vi "IRISS_FPGA_IO_v2.vi"() -> ()   [LabVIEW 2010]
doc: "This VI contains a basic quadrature decoder which is reset asynchronously upon clicking the reset button."
uses:
  <vilib>/platform/TimedLoop/XDataNode/XDataNode.xnode
  <vilib>/Platform/TimedLoop/XDataNode/nitl_modes.ctl
  <vilib>/Platform/TimedLoop/XDataNode/XDNodeRunTimeDep.lvlib
  <vilib>/Platform/TimedLoop/XDataNode/wakeup.ctl
  <vilib>/Platform/TimedLoop/XDataNode/timing_clust.ctl
  <vilib>/eio/EIONode/EIONode.xnode
  Library/KevinLibraryAll/labview/KevLib01.lvlib
panel:
  out "Home L4":bool
  out "Home L1":bool
  out "Home L2":bool
  out "Home L3":bool
  in  "Positive Direction C1-4":bool
  out "JumpBy2Error C1-4":i16
  out "32 bit Position C1-4":i32
  in  "Reset C1-4":bool
  in  "Positive Direction C1-1":bool
  out "JumpBy2Error C1-1":i16
  out "32 bit Position C1-1":i32
  in  "Reset C1-1":bool
  out "32 bit Position 17":i32
  in  "Reset 17":bool
  in  "Positive Direction 17":bool
  out "JumpBy2Error 17":i16
  out "32 bit Position 16":i32
  in  "Reset 16":bool
  in  "Positive Direction 16":bool
  out "JumpBy2Error 16":i16
  out "32 bit Position 15":i32
  in  "Reset 15":bool
  in  "Positive Direction 15":bool
  out "JumpBy2Error 15":i16
  out "32 bit Position 14":i32
  in  "Reset 14":bool
  in  "Positive Direction 14":bool
  out "JumpBy2Error 14":i16
  out "32 bit Position 13":i32
  in  "Reset 13":bool
  in  "Positive Direction 13":bool
  out "JumpBy2Error 13":i16
  out "32 bit Position 12":i32
  in  "Reset 12":bool
  in  "Positive Direction 12":bool
  out "JumpBy2Error 12":i16
  out "32 bit Position 11":i32
  in  "Reset 11":bool
  in  "Positive Direction 11":bool
  out "JumpBy2Error 11":i16
  out "32 bit Position 10":i32
  in  "Reset 10":bool
  in  "Positive Direction 10":bool
  out "JumpBy2Error 10":i16
  out "32 bit Position 9":i32
  in  "Reset 9":bool
  in  "Positive Direction 9":bool
  out "JumpBy2Error 9":i16
  out "JumpBy2Error 3":i16
  in  "Positive Direction 3":bool
  out "JumpBy2Error 1":i16
  in  "Positive Direction 1":bool
  out "AI":i16[](array[numeric])
  out "32 bit Position 3":i32
  in  "Reset 3":bool
  in  "AO":i16[](array[numeric])=[0, 0, 0, 0, 0, 0, 0, 0]
  out "32 bit Position 1":i32
  in  "Reset 1":bool
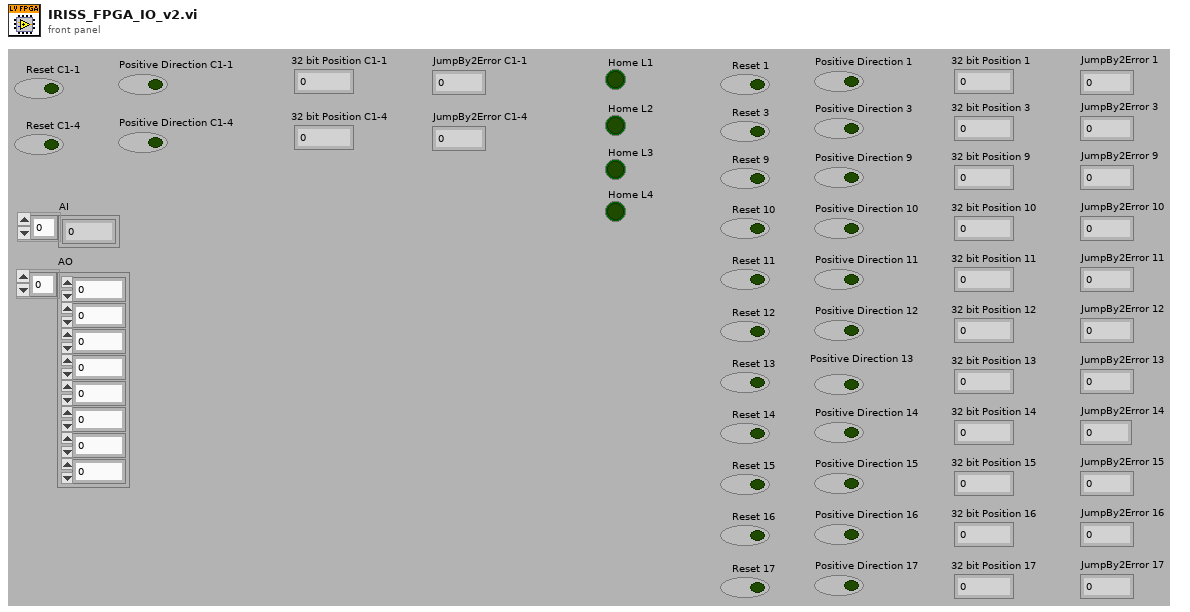
[diagram p1: front panel]
types:
  T1 = typedef "XDNodeRunTimeDep.lvlib/timing_clust.ctl" = cluster{"Expected End [f-1]":u64, "Actual End [f-1]":u64, "Finished Late? [f-1]":bool, "Expected End [i-1]":u64, "Actual End [i-1]":u64, "Finished Late? [i-1]":bool, "Expected Start [i]":u64, "Actual Start [i]":u64, "Expected Start [f]":u64, "Actual Start [f]":u64, "Source Name":string, "Structure Name":string, "Period":i64, "Deadline":i64, "Offset":i64, "Start":i64, "Priority":i32, "Timeout":i32, "Mode":T2, "Wakeup Reason":T3, "Error":errorcluster, "Source Type":string, "Secondary Source Type":string, "Global End Time":u64, "Global Start Time":u64, "Frame Duration":u64, "Iteration Duration":u64, "Assigned CPU":i32, "I/O Scan Engine Mode":u32}
  T2 = typedef "XDNodeRunTimeDep.lvlib/nitl_modes.ctl" = enum32{"No Change", "Process missed periods, maintain original phase", "Discard missed periods, maintain original phase", "Process missed periods, ignore original phase", "Discard missed periods, ignore original phase"}
  T3 = typedef "XDNodeRunTimeDep.lvlib/wakeup.ctl" = enum32{"Normal", "Aborted", "Asynchronous wakeup", "Timing source error", "Timed loop error", "Timeout"}
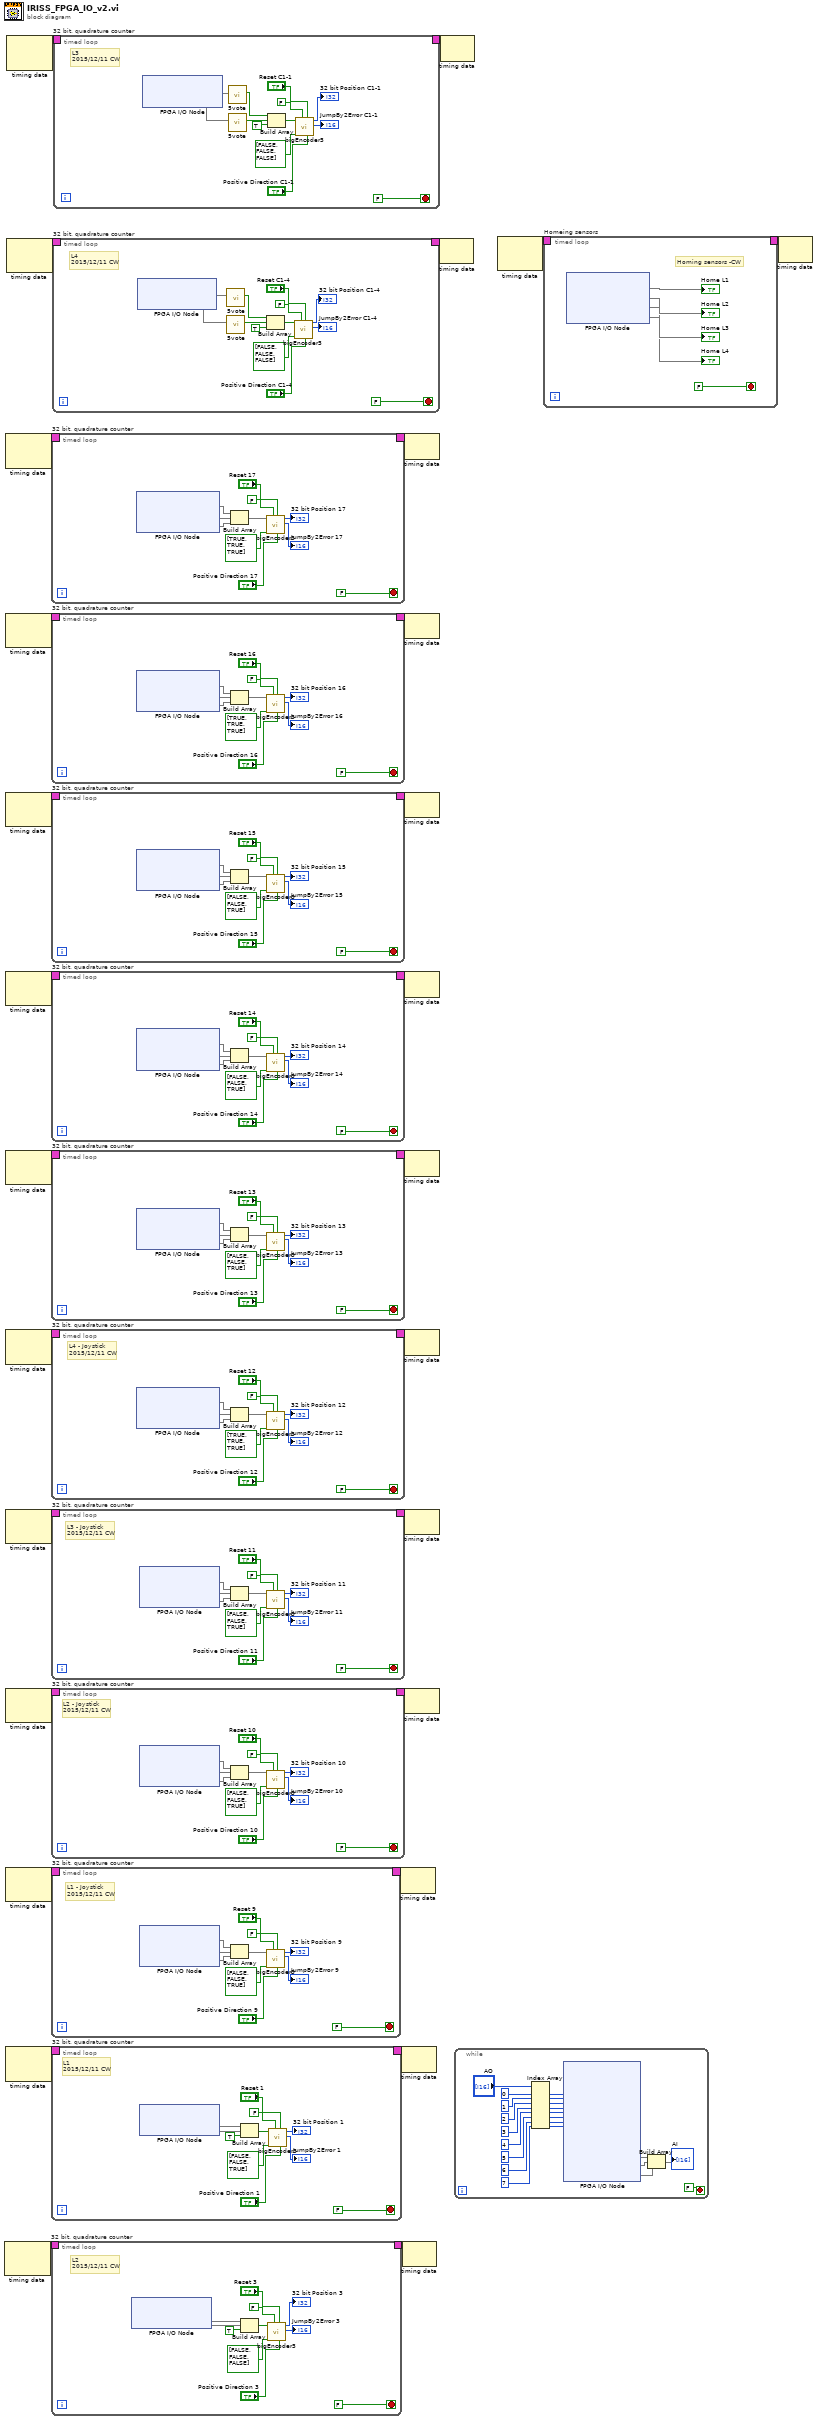
[diagram p0: block diagram]
diagram:
  n1 = node-c288() -> (w26:T1)  [unwired: 2 out]
  n2 = node-c288() -> (w8:T1)  [unwired: 2 out]
  n3 = node-c288() -> (w10:T1)  [unwired: 2 out]
  n4 = node-c288() -> (w12:T1)  [unwired: 2 out]
  n5 = node-c288() -> (w14:T1)  [unwired: 2 out]
  n6 = node-c288() -> (w16:T1)  [unwired: 2 out]
  n7 = node-c288() -> (w18:T1)  [unwired: 2 out]
  n8 = node-c288() -> (w20:T1)  [unwired: 2 out]
  n9 = node-c288() -> (w22:T1)  [unwired: 2 out]
  n10 = node-c288() -> (w24:T1)  [unwired: 2 out]
  n11 = node-c288() -> (w27:T1)  [unwired: 2 out]
  n12 = node-c288() -> (w4:T1)  [unwired: 2 out]
  n13 = node-c288() -> (w6:T1)  [unwired: 2 out]
  n14 = timed-loop "32 bit, quadrature counter" {
    timing-out: [_] -> w25
    timing: w26 -> [_]
    stop <- FALSE stop-if-true
    # "L2\n2015/12/11 CW"
    n15 = xnode "FPGA I/O Node"() -> ("Connector0/DIO2"=w32, "Connector0/DIO3"=w31)  [unwired: 2 in, 2 out]
    n16 = Build Array(w32, w31, TRUE ("element")) -> (w38:bool[])
    n17 = call "bigEncoder3.vi"("Positive Direction"="Positive Direction 3", "ForceReset"="Reset 3", "Allow C Reset?"=FALSE, "Reset Array"=bool[] [FALSE, FALSE, FALSE], "Encoder Array"=w38) -> ("JumpBy2Error"=→"JumpBy2Error 3":i16, "Position"=→"32 bit Position 3":i32)  [unwired: 5 out]
  }
  n18 = timed-loop "32 bit, quadrature counter" {
    timing-out: [_] -> w7
    timing: w8 -> [_]
    stop <- FALSE stop-if-true
    n19 = xnode "FPGA I/O Node"() -> ("Connector2/DIO24"=w51, "Connector2/DIO25"=w50, "Connector2/DIO26"=w42)  [unwired: 3 in, 3 out]
    n20 = Build Array(w51, w50, w42) -> (w49:void[])
    n21 = call "bigEncoder3.vi"("Positive Direction"="Positive Direction 17", "ForceReset"="Reset 17", "Allow C Reset?"=FALSE, "Reset Array"=bool[] [TRUE, TRUE, TRUE], "Encoder Array"=w49) -> ("JumpBy2Error"=→"JumpBy2Error 17":i16, "Position"=→"32 bit Position 17":i32)  [unwired: 5 out]
  }
  n22 = timed-loop "32 bit, quadrature counter" {
    timing-out: [_] -> w9
    timing: w10 -> [_]
    stop <- FALSE stop-if-true
    n23 = xnode "FPGA I/O Node"() -> ("Connector2/DIO21"=w64, "Connector2/DIO22"=w63, "Connector2/DIO23"=w55)  [unwired: 3 in, 3 out]
    n24 = Build Array(w64, w63, w55) -> (w62:void[])
    n25 = call "bigEncoder3.vi"("Positive Direction"="Positive Direction 16", "ForceReset"="Reset 16", "Allow C Reset?"=FALSE, "Reset Array"=bool[] [TRUE, TRUE, TRUE], "Encoder Array"=w62) -> ("JumpBy2Error"=→"JumpBy2Error 16":i16, "Position"=→"32 bit Position 16":i32)  [unwired: 5 out]
  }
  n26 = timed-loop "32 bit, quadrature counter" {
    timing-out: [_] -> w11
    timing: w12 -> [_]
    stop <- FALSE stop-if-true
    n27 = xnode "FPGA I/O Node"() -> ("Connector2/DIO18"=w77, "Connector2/DIO19"=w76, "Connector2/DIO20"=w68)  [unwired: 3 in, 3 out]
    n28 = Build Array(w77, w76, w68) -> (w75:void[])
    n29 = call "bigEncoder3.vi"("Positive Direction"="Positive Direction 15", "ForceReset"="Reset 15", "Allow C Reset?"=FALSE, "Reset Array"=bool[] [FALSE, FALSE, TRUE], "Encoder Array"=w75) -> ("JumpBy2Error"=→"JumpBy2Error 15":i16, "Position"=→"32 bit Position 15":i32)  [unwired: 5 out]
  }
  n30 = timed-loop "32 bit, quadrature counter" {
    timing-out: [_] -> w13
    timing: w14 -> [_]
    stop <- FALSE stop-if-true
    n31 = xnode "FPGA I/O Node"() -> ("Connector2/DIO15"=w90, "Connector2/DIO16"=w89, "Connector2/DIO17"=w81)  [unwired: 3 in, 3 out]
    n32 = Build Array(w90, w89, w81) -> (w88:void[])
    n33 = call "bigEncoder3.vi"("Positive Direction"="Positive Direction 14", "ForceReset"="Reset 14", "Allow C Reset?"=FALSE, "Reset Array"=bool[] [FALSE, FALSE, TRUE], "Encoder Array"=w88) -> ("JumpBy2Error"=→"JumpBy2Error 14":i16, "Position"=→"32 bit Position 14":i32)  [unwired: 5 out]
  }
  n34 = timed-loop "32 bit, quadrature counter" {
    timing-out: [_] -> w15
    timing: w16 -> [_]
    stop <- FALSE stop-if-true
    n35 = xnode "FPGA I/O Node"() -> ("Connector2/DIO12"=w103, "Connector2/DIO13"=w102, "Connector2/DIO14"=w94)  [unwired: 3 in, 3 out]
    n36 = Build Array(w103, w102, w94) -> (w101:void[])
    n37 = call "bigEncoder3.vi"("Positive Direction"="Positive Direction 13", "ForceReset"="Reset 13", "Allow C Reset?"=FALSE, "Reset Array"=bool[] [FALSE, FALSE, TRUE], "Encoder Array"=w101) -> ("JumpBy2Error"=→"JumpBy2Error 13":i16, "Position"=→"32 bit Position 13":i32)  [unwired: 5 out]
  }
  n38 = timed-loop "32 bit, quadrature counter" {
    timing-out: [_] -> w17
    timing: w18 -> [_]
    stop <- FALSE stop-if-true
    # "L4 - Joystick\n2015/12/11 CW"
    n39 = xnode "FPGA I/O Node"() -> ("Connector2/DIO9"=w116, "Connector2/DIO10"=w115, "Connector2/DIO11"=w107)  [unwired: 3 in, 3 out]
    n40 = Build Array(w116, w115, w107) -> (w114:void[])
    n41 = call "bigEncoder3.vi"("Positive Direction"="Positive Direction 12", "ForceReset"="Reset 12", "Allow C Reset?"=FALSE, "Reset Array"=bool[] [TRUE, TRUE, TRUE], "Encoder Array"=w114) -> ("JumpBy2Error"=→"JumpBy2Error 12":i16, "Position"=→"32 bit Position 12":i32)  [unwired: 5 out]
  }
  n42 = timed-loop "32 bit, quadrature counter" {
    timing-out: [_] -> w19
    timing: w20 -> [_]
    stop <- FALSE stop-if-true
    # "L3 - Joystick\n2015/12/11 CW"
    n43 = xnode "FPGA I/O Node"() -> ("Connector2/DIO6"=w129, "Connector2/DIO7"=w128, "Connector2/DIO8"=w120)  [unwired: 3 in, 3 out]
    n44 = Build Array(w129, w128, w120) -> (w127:void[])
    n45 = call "bigEncoder3.vi"("Positive Direction"="Positive Direction 11", "ForceReset"="Reset 11", "Allow C Reset?"=FALSE, "Reset Array"=bool[] [FALSE, FALSE, TRUE], "Encoder Array"=w127) -> ("JumpBy2Error"=→"JumpBy2Error 11":i16, "Position"=→"32 bit Position 11":i32)  [unwired: 5 out]
  }
  n46 = timed-loop "32 bit, quadrature counter" {
    timing-out: [_] -> w21
    timing: w22 -> [_]
    stop <- FALSE stop-if-true
    # "L2 - Joystick\n2015/12/11 CW"
    n47 = xnode "FPGA I/O Node"() -> ("Connector2/DIO3"=w142, "Connector2/DIO4"=w141, "Connector2/DIO5"=w133)  [unwired: 3 in, 3 out]
    n48 = Build Array(w142, w141, w133) -> (w140:void[])
    n49 = call "bigEncoder3.vi"("Positive Direction"="Positive Direction 10", "ForceReset"="Reset 10", "Allow C Reset?"=FALSE, "Reset Array"=bool[] [FALSE, FALSE, TRUE], "Encoder Array"=w140) -> ("JumpBy2Error"=→"JumpBy2Error 10":i16, "Position"=→"32 bit Position 10":i32)  [unwired: 5 out]
  }
  n50 = timed-loop "32 bit, quadrature counter" {
    timing-out: [_] -> w23
    timing: w24 -> [_]
    stop <- FALSE stop-if-true
    # "L1 - Joystick\n2015/12/11 CW"
    n51 = xnode "FPGA I/O Node"() -> ("Connector2/DIO0"=w155, "Connector2/DIO1"=w154, "Connector2/DIO2"=w146)  [unwired: 3 in, 3 out]
    n52 = Build Array(w155, w154, w146) -> (w153:void[])
    n53 = call "bigEncoder3.vi"("Positive Direction"="Positive Direction 9", "ForceReset"="Reset 9", "Allow C Reset?"=FALSE, "Reset Array"=bool[] [FALSE, FALSE, TRUE], "Encoder Array"=w153) -> ("JumpBy2Error"=→"JumpBy2Error 9":i16, "Position"=→"32 bit Position 9":i32)  [unwired: 5 out]
  }
  n54 = timed-loop "32 bit, quadrature counter" {
    timing-out: [_] -> w28
    timing: w27 -> [_]
    stop <- FALSE stop-if-true
    # "L1\n2015/12/11 CW"
    n55 = xnode "FPGA I/O Node"() -> ("Connector0/DIO0"=w168, "Connector0/DIO1"=w167)  [unwired: 2 in, 2 out]
    n56 = Build Array(w168, w167, TRUE ("element")) -> (w166:bool[])
    n57 = call "bigEncoder3.vi"("Positive Direction"="Positive Direction 1", "ForceReset"="Reset 1", "Allow C Reset?"=FALSE, "Reset Array"=bool[] [FALSE, FALSE, TRUE], "Encoder Array"=w166) -> ("JumpBy2Error"=→"JumpBy2Error 1":i16, "Position"=→"32 bit Position 1":i32)  [unwired: 5 out]
  }
  n58 = timed-loop "32 bit, quadrature counter" {
    timing-out: [_] -> w3
    timing: w4 -> [_]
    stop <- FALSE stop-if-true
    # "L4\n2015/12/11 CW"
    n59 = xnode "FPGA I/O Node"() -> ("Connector0/DIO6"=w175, "Connector0/DIO7"=w174)  [unwired: 2 in, 2 out]
    n60 = call "5vote.vi"("Input"=w175) -> ("vote5"=w172:bool)  [unwired: 10 in]
    n61 = call "5vote.vi"("Input"=w174) -> ("vote5"=w173:bool)  [unwired: 10 in]
    n62 = Build Array(w172, w173, TRUE ("element")) -> (w183:bool[])
    n63 = call "bigEncoder3.vi"("Positive Direction"="Positive Direction C1-4", "ForceReset"="Reset C1-4", "Allow C Reset?"=FALSE, "Reset Array"=bool[] [FALSE, FALSE, FALSE], "Encoder Array"=w183) -> ("JumpBy2Error"=→"JumpBy2Error C1-4":i16, "Position"=→"32 bit Position C1-4":i32)  [unwired: 5 out]
  }
  n64 = timed-loop "32 bit, quadrature counter" {
    timing-out: [_] -> w5
    timing: w6 -> [_]
    stop <- FALSE stop-if-true
    # "L3\n2015/12/11 CW"
    n65 = xnode "FPGA I/O Node"() -> ("Connector0/DIO4"=w190, "Connector0/DIO5"=w189)  [unwired: 2 in, 2 out]
    n66 = call "5vote.vi"("Input"=w190) -> ("vote5"=w187:bool)  [unwired: 10 in]
    n67 = call "5vote.vi"("Input"=w189) -> ("vote5"=w188:bool)  [unwired: 10 in]
    n68 = Build Array(w187, w188, TRUE ("element")) -> (w198:bool[])
    n69 = call "bigEncoder3.vi"("Positive Direction"="Positive Direction C1-1", "ForceReset"="Reset C1-1", "Allow C Reset?"=FALSE, "Reset Array"=bool[] [FALSE, FALSE, FALSE], "Encoder Array"=w198) -> ("JumpBy2Error"=→"JumpBy2Error C1-1":i16, "Position"=→"32 bit Position C1-1":i32)  [unwired: 5 out]
  }
  n70 = node-c288(w23) -> ()  [unwired: 1 out]
  n71 = node-c288(w28) -> ()  [unwired: 1 out]
  n72 = node-c288(w25) -> ()  [unwired: 1 out]
  n73 = node-c288(w7) -> ()  [unwired: 1 out]
  n74 = node-c288(w9) -> ()  [unwired: 1 out]
  n75 = node-c288(w11) -> ()  [unwired: 1 out]
  n76 = node-c288(w13) -> ()  [unwired: 1 out]
  n77 = node-c288(w15) -> ()  [unwired: 1 out]
  n78 = node-c288(w17) -> ()  [unwired: 1 out]
  n79 = node-c288(w19) -> ()  [unwired: 1 out]
  n80 = node-c288(w21) -> ()  [unwired: 1 out]
  n81 = node-c288(w3) -> ()  [unwired: 1 out]
  n82 = node-c288(w5) -> ()  [unwired: 1 out]
  n83 = while {
    stop <- FALSE stop-if-true
    n84 = Index Array(array="AO", index #1=0 ("index"), index #2=1 ("index"), index #3=2 ("index"), index #4=3 ("index"), index #5=4 ("index"), index #6=5 ("index"), index #7=6 ("index"), index #8=7 ("index")) -> (element #1=w214:i16, element #2=w213:i16, element #3=w212:i16, element #4=w211:i16, element #5=w210:i16, element #6=w209:i16, element #7=w208:i16, element #8=w207:i16)
    n85 = xnode "FPGA I/O Node"("Connector0/AO0"=w214, "Connector0/AO1"=w213, "Connector0/AO2"=w212, "Connector0/AO3"=w211, "Connector0/AO4"=w210, "Connector0/AO5"=w209, "Connector0/AO6"=w208, "Connector0/AO7"=w207) -> ("Connector0/AI0"=w205, "Connector0/AI1"=w204, "Connector0/AI2"=w202)  [unwired: 11 in, 11 out]
    n86 = Build Array(w205, w204, w202) -> (→"AI":void[])
  }
  n87 = node-c288() -> (w2:T1)  [unwired: 2 out]
  n88 = timed-loop "Homeing sensors" {
    timing-out: [_] -> w1
    timing: w2 -> [_]
    stop <- FALSE stop-if-true
    # "Homing sensors -CW"
    n89 = xnode "FPGA I/O Node"() -> ("Connector0/DIO8"=→"Home L1", "Connector0/DIO9"=→"Home L2", "Connector0/DIO10"=→"Home L3", "Connector0/DIO11"=→"Home L4")  [unwired: 4 in, 4 out]
  }
  n90 = node-c288(w1) -> ()  [unwired: 1 out]
